vi "Homing.vi"() -> (3 "Final de Carrera":bool)   [LabVIEW 2017]
panel:
  in  "Home":bool
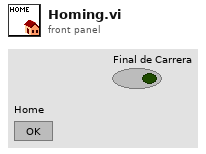
[diagram p1: front panel]
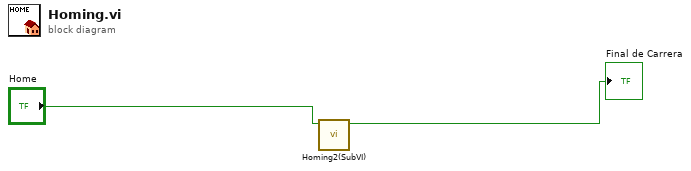
[diagram p0: block diagram]
diagram:
  n1 = call "Homing2(SubVI).vi"("Home"="Home") -> ("Boolean"=→"Final de Carrera":bool)  [unwired: 10 in]
